vi "Transmit Message Dynamic.vi"(8 "error in (no error)":errorcluster, 10 "message data":u32 format="%08x", 11 "channel handle in":u64) -> (0 "error out":errorcluster, 3 "channel handle out":u64)   [LabVIEW 2020, in "Ballard ARINC 429 Hardware API.lvlib"]
doc: "Appends a dynamically defined message to the asynchronous list buffer. Data already in the buffer will not be removed.\n\nThe asynchronous list buffer attempts to transmit data within its buffer when gaps of 36 bit times or more are encountered in the transmission schedule of the channel. It allows for easy definition of dynamic data on the channel without interrupting existing scheduled label transmission rates.\n\nIf the <B>asyncMessageList</B> node is not defined by the configuration file, this VI will return an error."
uses:
  Ballard ARINC 429 Hardware API.lvlib
  BTI429LV.dll
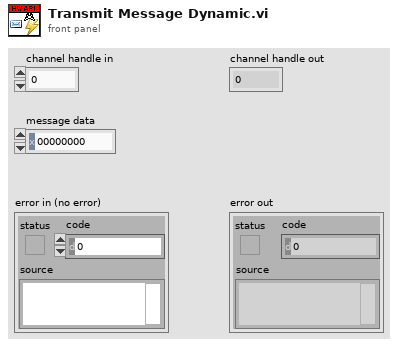
[diagram p1: front panel]
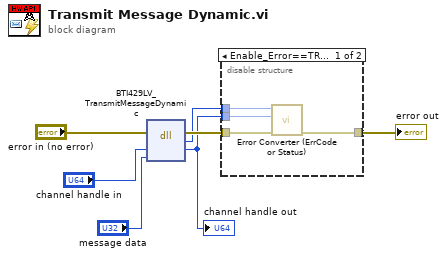
[diagram p0: block diagram]
diagram:
  n1 = dll-call lib="BTI429LV.*" fn="BTI429LV_TransmitMessageDynamic"(error in="error in (no error)", "chanhandle"="channel handle in", "value"="message data") -> (error out=w4:errorcluster, "return type"=w3:i32, "chanhandle"=w2:u64)  [unwired: 3 in, 1 out]
  "channel handle out" <- w2
  n2 = disable-structure shown="Enable_Error==TRUE" {
    disable-tunnel: w4 -> [w11 w12]
    disable-tunnel: [w10 w12] -> w1
    disable-tunnel: w3 -> [w9 _]
    disable-tunnel: w2 -> [w8 _]
    frame condition #0 {
      n3 = call "Error Converter (ErrCode or Status).vi"("error in (no error)"=w11, "handle in"=w8, "error code"=w9) -> ("error out"=w10:errorcluster)  [unwired: 8 in]
    }
    frame condition #1 (active) {
    }
  }
  "error out" <- w1
